vi "MSControlSuite_main.vi"() -> ()   [LabVIEW 2015]
doc: "This is the main program/main menu for the whole MSControl Suite."
panel:
  in  "Setup Button":bool
  in  "MSEval Button":bool
  in  "MSControl Button":bool
  # "MS Control Suite"
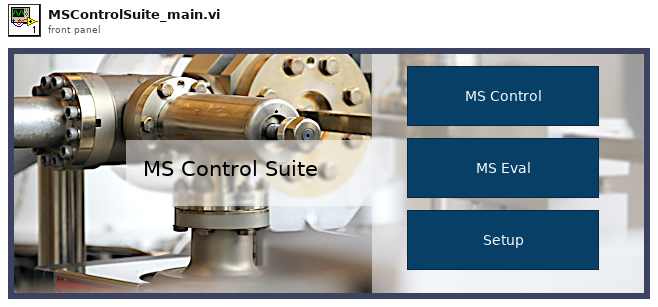
[diagram p1: front panel]
types:
  T1 = enum32{"Invalid", "Standard", "Closed", "Hidden", "Minimized", "Maximized"}
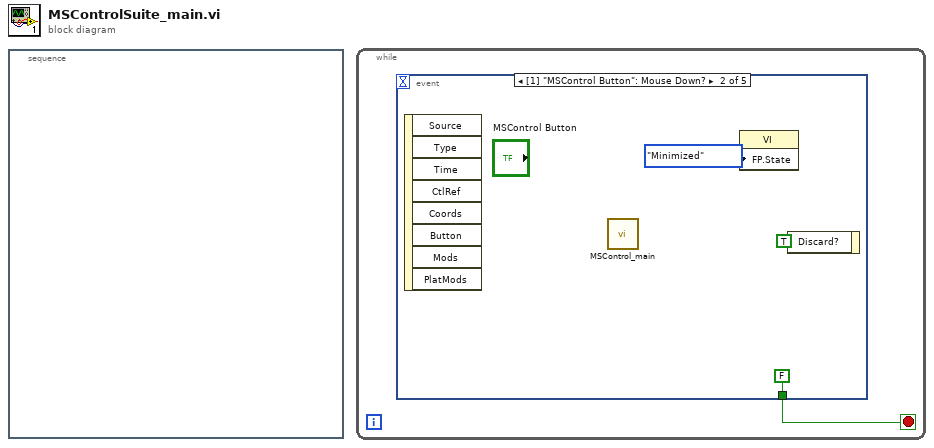
[diagram p0: block diagram]
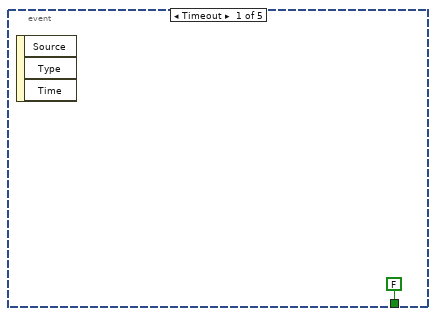
[diagram p2: hidden frame]
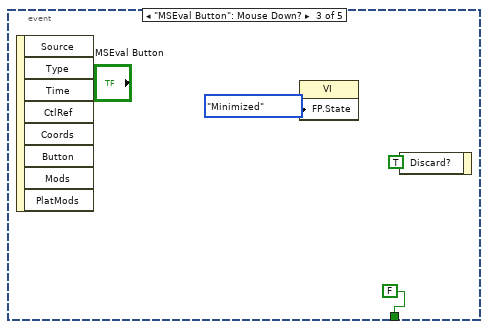
[diagram p3: hidden frame]
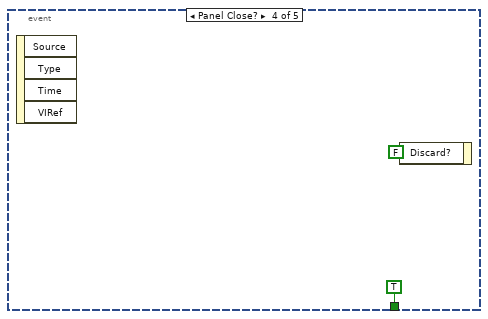
[diagram p4: hidden frame]
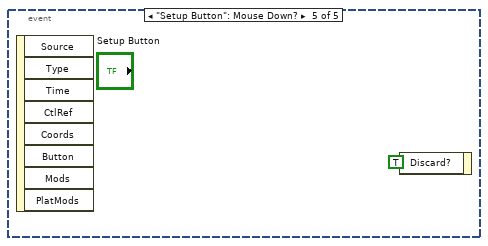
[diagram p5: hidden frame]
diagram:
  n1 = stacked-sequence {
    frame #0 {
    }
  }
  n2 = while {
    stop <- w1 stop-if-true
    n3 = event shown="[1] \"MSControl Button\": Mouse Down?" {
      selector: _ -> [_ _ _ _ _]
      dyn-events: _ -> [_ _ _ _ _]
      timeout: _ -> [_ _ _ _ _]
      tunnel: [FALSE FALSE FALSE TRUE _] -> w1
      event Timeout {
        n4 = event-data() -> ()  [unwired: 1 in, 3 out]
      }
      event "MSControl Button": Mouse Down? {
        n5 = event-data() -> ()  [unwired: 1 in, 8 out]
        n6 = call "MSControl_main.vi"() -> ()  [unwired: 12 in]
        n7 = property class="VI"("FP.State"=T1."Minimized" ("Front Panel Window:State")) -> ()  [unwired: 2 in, 2 out]
        n8 = event-data("Discard?"=TRUE) -> ()  [unwired: 1 in, 1 out]
      }
      event "MSEval Button": Mouse Down? {
        n9 = event-data() -> ()  [unwired: 1 in, 8 out]
        n10 = property class="VI"("FP.State"=T1."Minimized" ("Front Panel Window:State")) -> ()  [unwired: 2 in, 2 out]
        n11 = event-data("Discard?"=TRUE) -> ()  [unwired: 1 in, 1 out]
      }
      event Panel Close? {
        n12 = event-data() -> ()  [unwired: 1 in, 4 out]
        n13 = event-data("Discard?"=FALSE) -> ()  [unwired: 1 in, 1 out]
      }
      event "Setup Button": Mouse Down? {
        n14 = event-data() -> ()  [unwired: 1 in, 8 out]
        n15 = event-data("Discard?"=TRUE) -> ()  [unwired: 1 in, 1 out]
      }
    }
  }
